vi "Network Steam Read Message.vi"(6 "Timeout(ms)":i32, 8 "error in (no error)":errorcluster, 11 "Model in":refnum<class "Model.lvclass">) -> (0 "error out":errorcluster, 1 "Message":T1, 2 "StillConnected?":bool, 3 "Model out":refnum<class "Model.lvclass">, 4 "Timed Out?":bool)   [LabVIEW 2021, in "Model.lvlib" / "Model.lvclass"]
uses:
  Model.lvclass
  Model.lvclass/Model.ctl
  <userlib>/John_Lib/Network_Streams_Connection/NetworkConnection.lvclass
  <userlib>/John_Lib/Network_Streams_Connection/NetworkCommand--Cluster.ctl
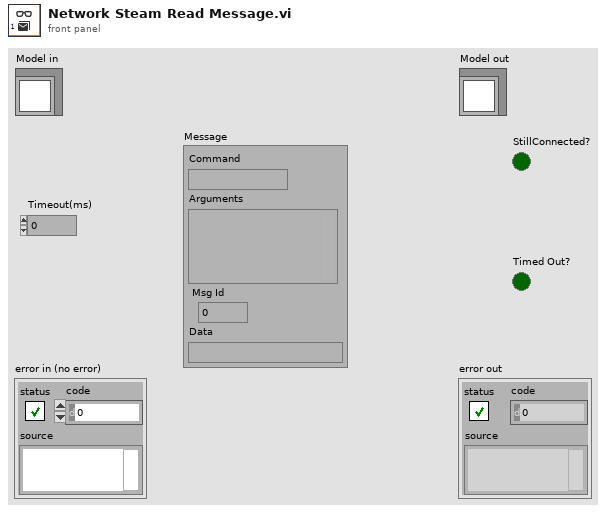
[diagram p1: front panel]
types:
  T1 = typedef "JKI_Network_Streams.lvlib/NetworkConnection.lvclass/NetworkCommand--Cluster.ctl" = cluster{"Command":string, "Arguments":variant, " Msg Id":i32, "Data":string}
  T2 = typedef "Model.lvlib/Model.lvclass/DVR.ctl" = cluster{"JKI_Network_Streams":refnum<class "NetworkConnection.lvclass">}
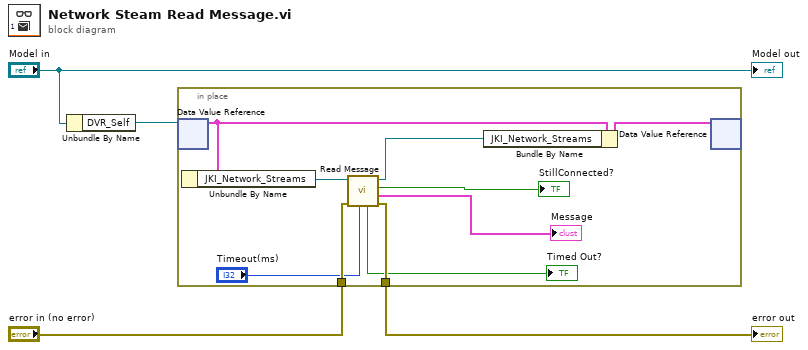
[diagram p0: block diagram]
diagram:
  n1 = Unbundle By Name("Model in") -> ("DVR_Self"=w3:refnum<data-value>)
  n2 = in-place {
    in-place-border: "error in (no error)" -> [w10]
    in-place-border: [w8] -> w1
    n3 = in-place-dvr #1(w3) -> (w14:T2)  [unwired: 1 out]
    n4 = Unbundle By Name(w14) -> ("JKI_Network_Streams"=w13:refnum<class "NetworkConnection.lvclass">)
    n5 = call <userlib>:"Read Message.vi"("Timeout(ms)"="Timeout(ms)", "error in (no error)"=w10, "NetworkConnection in"=w13) -> ("error out"=w8:errorcluster, "Message"=→"Message":T1, "StillConnected?"=→"StillConnected?":bool, "NetworkConnection out"=w11:refnum<class "NetworkConnection.lvclass">, "Timed Out?"=→"Timed Out?":bool)  [unwired: 3 in, 1 out]
    n6 = Bundle By Name(cluster=w14, "JKI_Network_Streams"=w11) -> (w12:T2)
    n7 = in-place-dvr #1(w12) -> ()  [unwired: 2 out]
  }
  "error out" <- w1
  "Model out" <- "Model in"
